vi "Queue Message Handle Create.vi"(6 "Data Path":path, 7 "Project Name":string, 8 "error in (no error)":errorcluster caption="Error In", 9 "Name":string, 10 "Title":string, 11 "Queue Ref In":T1={"UI"=refnum, "Message"=refnum, "Data"=refnum, "Caller"=refnum, "Name"="000 Common", "Data Path"=path "", "Class Path"=path "", "SubPanel"=refnum, "Project Name"="", "MNT"="", "Title"="", "Data Source"=refnum, "Queue List"={}, "VI"=refnum, "UE"=refnum}) -> (0 "error out":errorcluster caption="Error Out", 3 "Queue Ref Out":T1={"UI"=refnum, "Message"=refnum, "Data"=refnum, "Caller"=refnum, "Name"="000 Common", "Data Path"=path "", "Class Path"=path "", "SubPanel"=refnum, "Project Name"="", "MNT"="", "Title"="", "Data Source"=refnum, "Queue List"={}, "VI"=refnum, "UE"=refnum}, 5 "call chain":string[](array[string]))   [LabVIEW 2020]
uses:
  000 Module Data Type.ctl
  Queue Message.ctl
  Modules/9999 SubVI/Global/Data Global/Data Global Mode.ctl
  Modules/006 Path Management/006 System Gloabl.vi
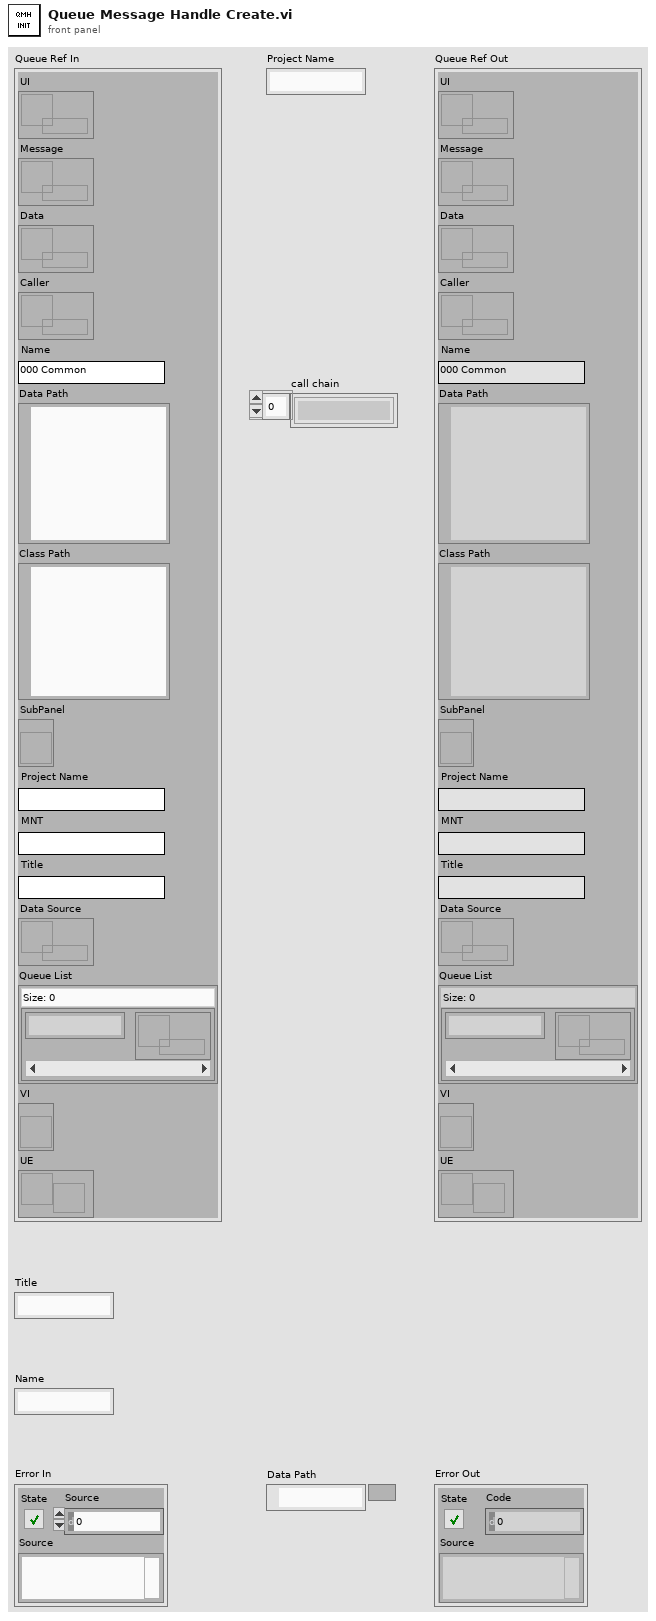
[diagram p1: front panel]
types:
  T1 = typedef "000 Module Data Type.ctl" = cluster{"UI":refnum<queue>, "Message":refnum<queue>, "Data":refnum<queue>, "Caller":refnum<queue>, "Name":string, "Data Path":path, "Class Path":path, "SubPanel":refnum<vi>, "Project Name":string, "MNT":string, "Title":string, "Data Source":refnum<queue>, "Queue List":map{string, refnum<queue>}, "VI":refnum<vi>, "UE":refnum<user-event>}
  T2 = typedef "Data Global Mode.ctl" = enum16{"Init", "Read", "Write", "Write Data", "Load"}
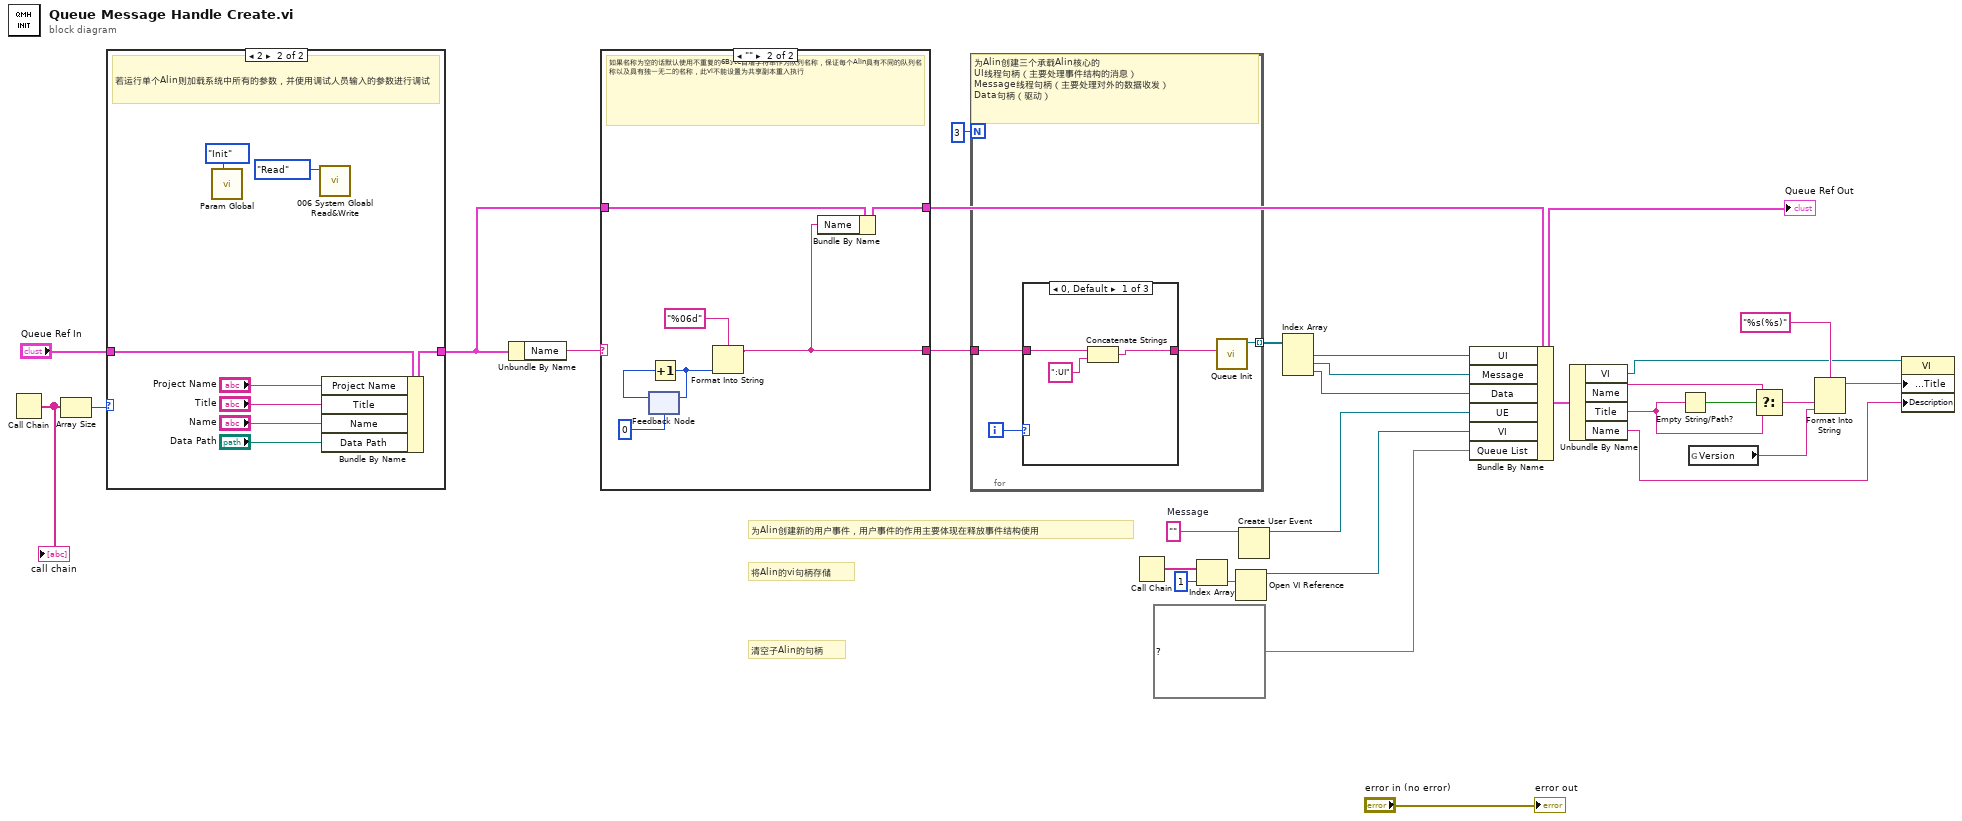
[diagram p0: block diagram]
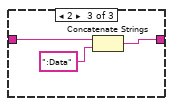
[diagram p3: hidden frame]
diagram:
  w16 = ""  # Message
  # "为Alin创建新的用户事件，用户事件的作用主要体现在释放事件结构使用"
  # "将Alin的vi句柄存储"
  # "清空子Alin的句柄"
  n1 = Call Chain() -> (call chain=w19:string[])
  "call chain" <- w19
  n2 = Array Size(array=w19) -> (size(s)=w18:i32)
  n3 = case shown="2" w18 {
    tunnel: "Queue Ref In" -> [w31 w39]
    tunnel: [w31 w38] -> w2
    frame 3.., Default {
      # "默认执行此分支，所有的默认属性有父Alin指定"
    }
    frame 2 {
      # "若运行单个Alin则加载系统中所有的参数，并使用调试人员输入的参数进行调试"
      n4 = call "Param Global.vi"("Operate"=Data_Global_Mode."Init") -> ()  [unwired: 9 in, 2 out]
      n5 = call "006 System Gloabl Read&Write.vi"("RW"=enum16{"Read", "Write"}."Read") -> ()  [unwired: 7 in, 4 out]
      n6 = Bundle By Name(cluster=w39, "Project Name"="Project Name", "Title"="Title", "Name"="Name", "Data Path"="Data Path") -> (w38:T1)
    }
  }
  n7 = Unbundle By Name(w2) -> ("Name"=w4:string)
  n8 = case shown="\"\"" w4 {
    selector: w4 -> [w41 _]
    tunnel: [w41 w42] -> w3
    tunnel: w2 -> [w40 w44]
    tunnel: [w40 w43] -> w1
    frame Default {
    }
    frame "" {
      # "如果名称为空的话默认使用不重复的6Byte自增字符串作为队列名称，保证每个Alin具有不同的队列名称以及具有独一无二的名称，此vi不能设置为共享副本重入执行"
      n9 = feedback #1(u32 0) -> (w47:u32)
      n10 = Increment(x=w47) -> (x+1=w48:u32)
      n11 = feedback-in #1(w48) -> ()
      n12 = Format Into String(format string="%06d" ("格式字符串"), w48) -> (resulting string=w42:string)  [unwired: 2 in, 1 out]
      n13 = Bundle By Name(cluster=w44, "Name"=w42) -> (w43:T1)
    }
  }
  n14 = for {
    N: 3 -> [_]
    tunnel: [w52] -> w30 mode=indexing
    tunnel: w3 -> [w49]
    i -> [w50]
    # "为Alin创建三个承载Alin核心的\nUI线程句柄（主要处理事件结构的消息）\nMessage线程句柄（主要处理对外的数据收发）\nData句柄（驱动）"
    n15 = case shown="0, Default" w50 {
      tunnel: [w53 w56 w57] -> w51
      tunnel: w49 -> [w55 w56 w58]
      frame 0, Default {
        n16 = Concatenate Strings(w55, ":UI" ("字符串")) -> (w53:string)
      }
      frame 1 {
      }
      frame 2 {
        n17 = Concatenate Strings(w58, ":Data" ("字符串")) -> (w57:string)
      }
    }
    n18 = call "Queue Init.vi"("Queue Name"=w51) -> ("Queue Out"=w52:refnum<queue>)  [unwired: 8 in, 2 out]
  }
  n19 = Call Chain() -> (call chain=w14:string[])
  n20 = Index Array(array=w14, index=1 ("索引")) -> (element=w13:string)
  n21 = Open VI Reference(vi path=w13) -> (vi reference=w11:refnum<vi>)  [unwired: 5 in, 1 out]
  n22 = Create User Event(user event datatype=w16) -> (user event=w12:refnum<user-event>)  [unwired: 1 in, 1 out]
  n23 = Index Array(array=w30) -> (element #1=w28:refnum<queue>, element #2=w5:refnum<queue>, element #3=w27:refnum<queue>)  [unwired: 3 in]
  n24 = Bundle By Name(cluster=w1, "UI"=w28, "Message"=w5, "Data"=w27, "UE"=w12, "VI"=w11, "Queue List"=map{string, refnum<queue>} {}) -> (w7:T1)
  "Queue Ref Out" <- w7
  n25 = Unbundle By Name(w7) -> ("VI"=w10:refnum<vi>, "Name"=w22:string, "Title"=w9:string, "Name"=w8:string)
  n26 = Empty String/Path?(string/path=w9) -> (empty?=w23:bool)
  n27 = global read "006 System Gloabl.vi" "Version"() -> (w24:string)
  n28 = Select(t=w22, s=w23, f=w9) -> (s? t:f=w21:string)
  n29 = Format Into String(format string="%s(%s)" ("格式字符串"), w21, w24) -> (resulting string=w20:string)  [unwired: 2 in, 1 out]
  n30 = property class="VI"(reference=w10, "Front Panel.Title"=w20, "Description"=w8) -> ()  [unwired: 1 in, 2 out]
  "error out" <- "error in (no error)"
